vi "Write Thrust Allocation Matrix.vi"(8 "error in (no error)":errorcluster, 10 "Real Matrix":T1, 11 "Thrust Allocation in":refnum<class "Thrust Allocation.lvclass">) -> (0 "error out":errorcluster, 3 "Thrust Allocation out":refnum<class "Thrust Allocation.lvclass">)   [LabVIEW 2014, in "Thrust Allocation.lvclass"]
uses:
  Thrust Allocation.lvclass
  <vilib>/Analysis/Matrix/Datatypes/RealMatrix.ctl
  Thrust Allocation.lvclass/Thrust Allocation.ctl
  <vilib>/Analysis/Matrix/NI_Matrix.lvlib
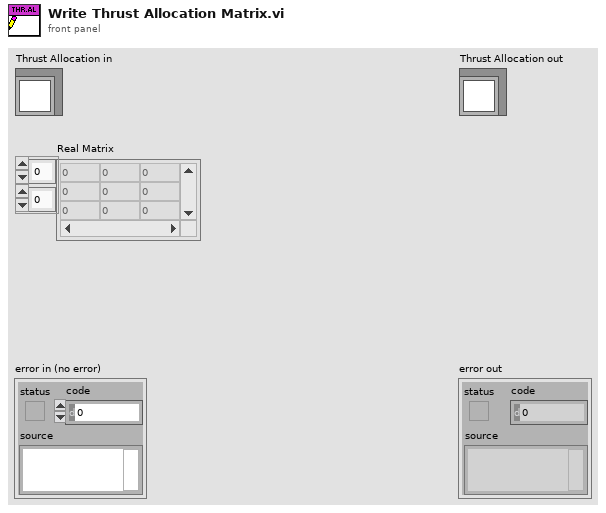
[diagram p1: front panel]
types:
  T1 = typedef "NI_Matrix.lvlib/RealMatrix.ctl" = dbl[][]
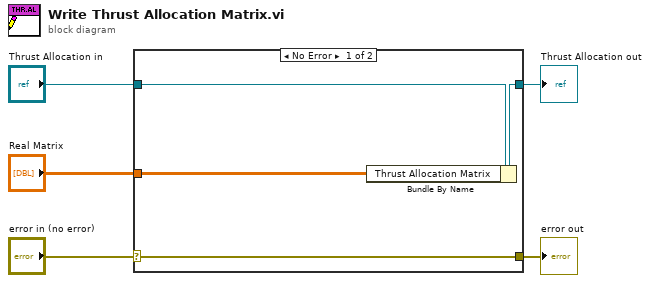
[diagram p0: block diagram]
diagram:
  n1 = case shown="No Error" "error in (no error)" {
    selector: "error in (no error)" -> [w9 w10]
    tunnel: [w9 w10] -> w4
    tunnel: [w7 w11] -> w2
    tunnel: "Thrust Allocation in" -> [w8 w11]
    tunnel: "Real Matrix" -> [w6 _]
    frame No Error {
      n2 = Bundle By Name(cluster=w8, "Thrust Allocation Matrix"=w6) -> (w7:refnum<class "Thrust Allocation.lvclass">)
    }
    frame Error {
    }
  }
  "error out" <- w4
  "Thrust Allocation out" <- w2
